vi "IsValid2001.vi"   [LabVIEW 2013]
uses:
  <vilib>/Heliosphere Research LLC/Advanced Plotting Toolkit/typedefs/PlotID.ctl
  <vilib>/Heliosphere Research LLC/Advanced Plotting Toolkit/Advanced Plotting Toolkit.lvlib
types:
  T1 = typedef "Advanced Plotting Toolkit.lvlib/PlotID.ctl" = i32
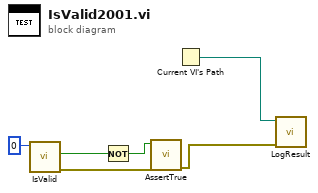
[diagram p0: block diagram]
diagram:
  n1 = call <vilib>:"IsValid.vi"("Plot ID"=T1 0) -> ("error out"=w5:errorcluster, "Valid?"=w2:bool)  [unwired: 8 in, 1 out]
  n2 = Not(x=w2) -> (.not. x?=w1:bool)
  n3 = call "AssertTrue.vi"("error in (no error)"=w5, "Value"=w1) -> ("error out"=w4:errorcluster)  [unwired: 9 in]
  n4 = Current VI's Path() -> (path=w6:path)
  n5 = call "LogResult.vi"("Test Result"=w4, "VI Path"=w6) -> ()  [unwired: 10 in]
